vi "CST_Reg_CHxSET.vi"() -> (0 "CH1SET":T1={"PD#"=enum."Normal Operation", "GAIN#"=enum."6", "SRB2"=enum."Open (Off)", "MUX#"=enum."Normal Electrode"})   [LabVIEW 2010]
uses:
  Controls/Register/TYP_Reg_CHxSET.ctl
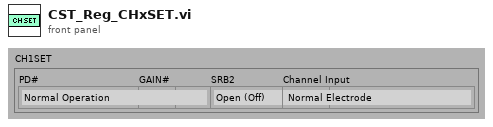
[diagram p1: front panel]
types:
  T1 = typedef "TYP_Reg_CHxSET.ctl" = cluster{"PD#":enum16{"Normal Operation", "Power-down"}, "GAIN#":enum16{"1", "2", "4", "6", "8", "12", "24"}, "SRB2":enum16{"Open (Off)", "Closed (On)"}, "MUX#":enum16{"Normal Electrode", "Input Short", "BIAS Measurement", "MVDD", "Temperature Sensor", "Test Signal", "BIAS Positive Electrode Driver", "BIAS Negative Electrode Driver"}}
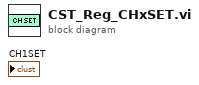
[diagram p0: block diagram]
diagram:
